vi "pp2_log_state.vi"(8 "Log memo?":bool, 10 "refnum in":refnum<file>, 11 "State In":T1={"Curr  tr"=0, "Curr (ms)"=0, "Cum (ms)"=0, "Run loop diff"=0, "Tone countdown (ms)"=0, "Countdown (ms)"=0, "Curr State"=enum."0 NULL", "Prev State"=enum."1 Habituation", "Null"=FALSE, "Sw"=FALSE, "Tone\nGate"=FALSE, "Stim"=FALSE, "Current DAQ DO Int"=0, "Current Loaded Trial"={"Trial Type Number"=1, "Trial Type"=enum."GO", "Trial Weight"=100, "Shock (mA)"=0.3, "Duration (ms)"=0.25, "Sound Type"=enum."04 FM Sweep", "Stim P1"=4000.0, "Stim P2"=0.0, "Stim P3"=0.0, "Stim P4"=2000.0}, "Next Trial (for display purposes)"={"Trial Type Number"=1, "Trial Type"=enum."GO", "Trial Weight"=100, "Shock (mA)"=0.3, "Duration (ms)"=0.25, "Sound Type"=enum."04 FM Sweep", "Stim P1"=4000.0, "Stim P2"=0.0, "Stim P3"=0.0, "Stim P4"=2000.0}, "Total trials memo"=0, "State start cum memo (ms)"=0, "Last dur jump time memo (ms)"=0, "Last dur shock time memo (ms)"=0, "Tone repeat memo (ms)"=0, "Webcam on"=FALSE, "Webcam recording"=FALSE} {"Current DAQ DO Int" format="%b"; "Next Trial (for display purposes)"."Shock (mA)" min=-1.0 max=5.0; "Next Trial (for display purposes)"."Trial Weight" step=1; "Next Trial (for display purposes)"."Duration (ms)" min=0.0 max=1.0; "Next Trial (for display purposes)"."Trial Type Number" min=1 step=1; "Current Loaded Trial"."Shock (mA)" min=-1.0 max=5.0; "Current Loaded Trial"."Trial Weight" step=1; "Current Loaded Trial"."Duration (ms)" min=0.0 max=1.0; "Current Loaded Trial"."Trial Type Number" min=1 step=1}) -> (2 "refnum out":refnum<file>)   [LabVIEW 2013]
uses:
  pp2_CTL_StateInfo.ctl
  pp2_CTL_State.ctl
  pp2_Trial.ctl
  pp2_CTL_TrialType.ctl
  labolabo2/waveforms/WFTypes.ctl
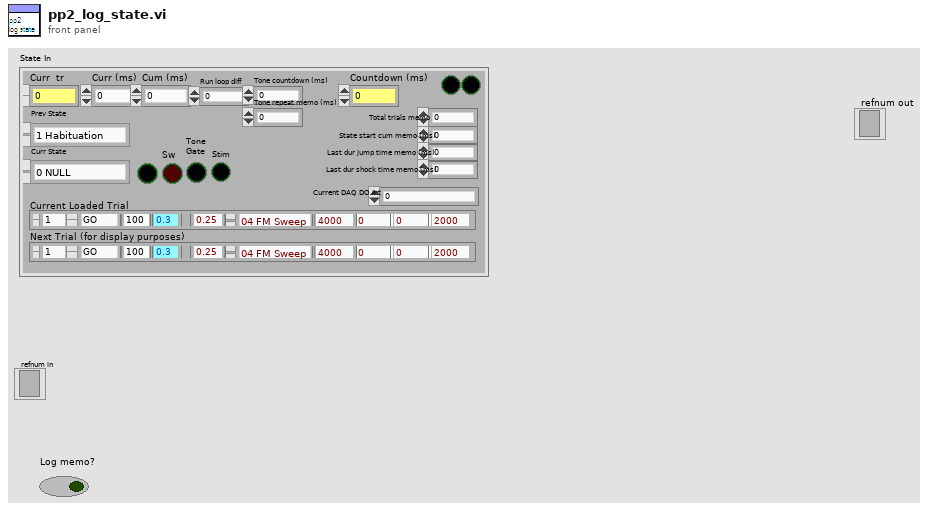
[diagram p1: front panel]
types:
  T1 = typedef "pp2_CTL_StateInfo.ctl" = cluster{"Curr  tr":u16, "Curr (ms)":u32, "Cum (ms)":i64, "Run loop diff":i64, "Tone countdown (ms)":i64, "Countdown (ms)":i64, "Curr State":T2, "Prev State":T2, "Null":bool, "Sw":bool, "Tone\nGate":bool, "Stim":bool, "Current DAQ DO Int":u16, "Current Loaded Trial":T3, "Next Trial (for display purposes)":T3, "Total trials memo":i64, "State start cum memo (ms)":i64, "Last dur jump time memo (ms)":i64, "Last dur shock time memo (ms)":i64, "Tone repeat memo (ms)":i64, "Webcam on":bool, "Webcam recording":bool}
  T2 = typedef "pp2_CTL_State.ctl" = enum8{"0 NULL", "1 Habituation", "2 (Load Trial)", "3 Stay Period", "4 Load Audio/Click Delay", "5 GO Trial", "6 GO Jumped", "7 GO Timeout", "8 NOGO Trial", "9 NOGO Jumped", "10 NOGO Timeout", "11 TEST Trial", "12 TEST Jumped", "13 TEST Timeout", "14 Intertrial Interval", "15 Done"}
  T3 = typedef "pp2_Trial.ctl" = cluster{"Trial Type Number":u8, "Trial Type":T4, "Trial Weight":u32, "Shock (mA)":dbl, "Duration (ms)":dbl, "Sound Type":T5, "Stim P1":dbl, "Stim P2":dbl, "Stim P3":dbl, "Stim P4":dbl}
  T4 = typedef "pp2_CTL_TrialType.ctl" = enum16{"OFF", "GO", "NOGO", "TEST"}
  T5 = typedef "WFTypes.ctl" = enum16{"00 NULL", "01 DC", "02 Noise", "03 Pure Tone", "04 FM Sweep"}
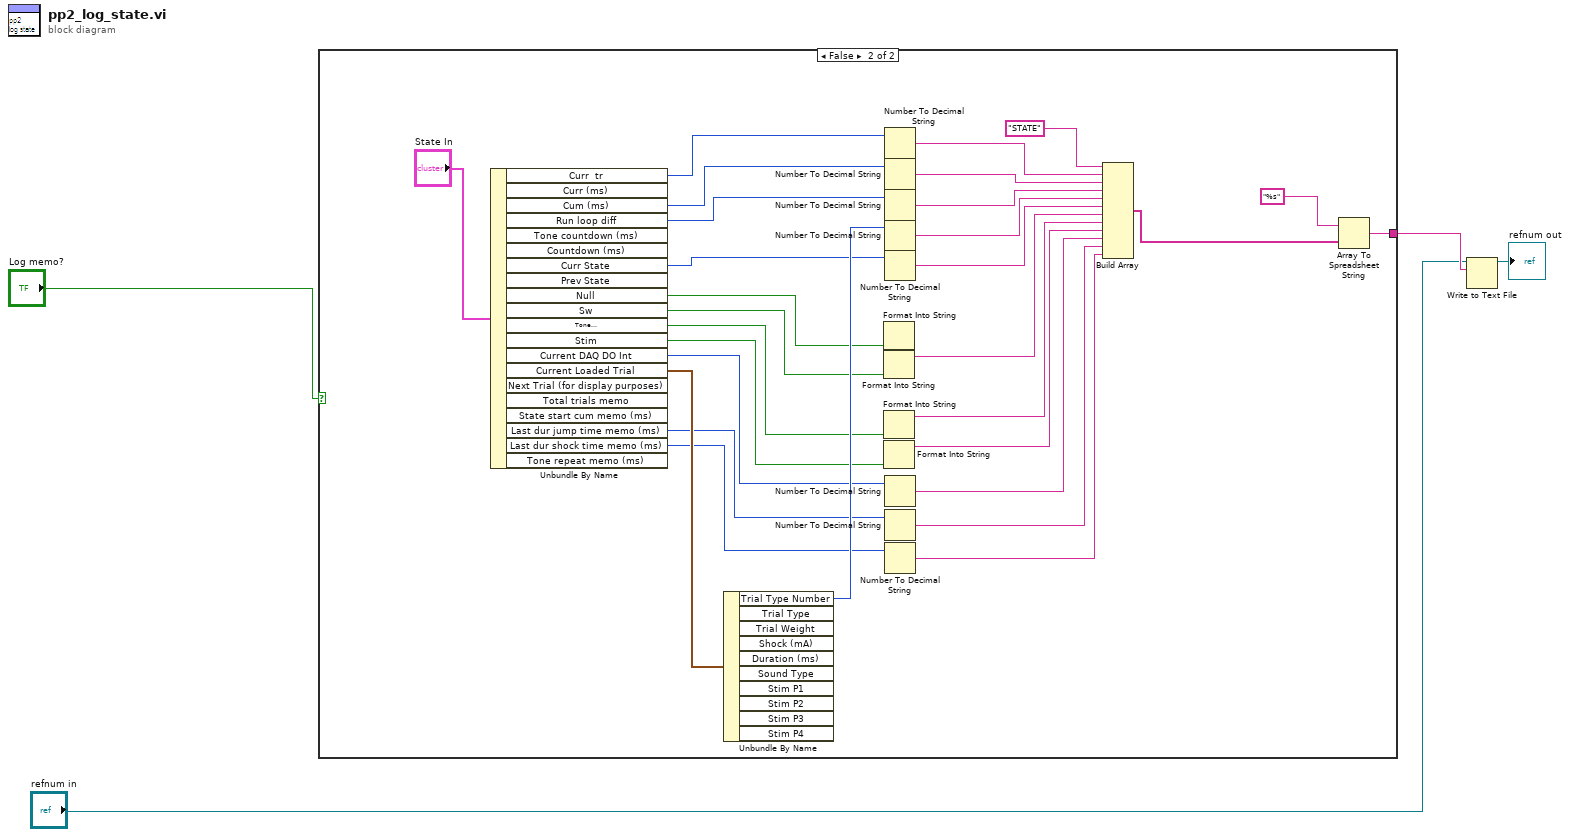
[diagram p0: block diagram]
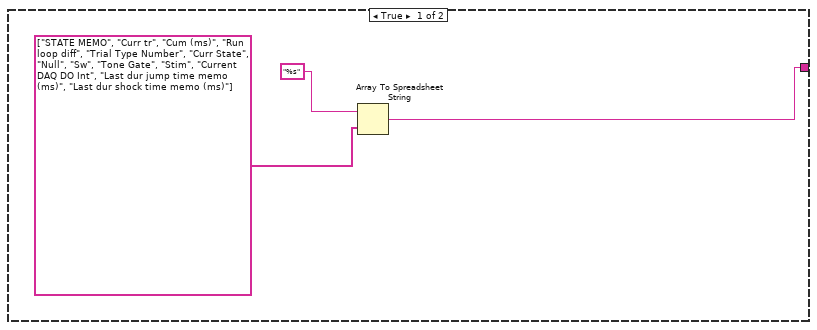
[diagram p2: hidden frame]
diagram:
  n1 = case shown="False" "Log memo?" {
    tunnel: [w5 w29] -> w4
    frame True {
      n2 = Array To Spreadsheet String(array=string[] ["STATE MEMO", "Curr tr", "Cum (ms)", "Run loop diff", "Trial Type Number", "Curr State", "Null", "Sw", "Tone Gate", "Stim", "Current DAQ DO Int", "Last dur jump time memo (ms)", "Last dur shock time memo (ms)"], 3:"%s" ("format string")) -> (spreadsheet string=w5:string)  [unwired: 1 in]
    }
    frame False {
      n3 = Unbundle By Name("State In") -> ("Curr  tr"=w26:u16, "Cum (ms)"=w25:i64, "Run loop diff"=w24:i64, "Curr State"=w21:T2, "Null"=w20:bool, "Sw"=w19:bool, "Tone\nGate"=w18:bool, "Stim"=w17:bool, "Current DAQ DO Int"=w8:u16, "Current Loaded Trial"=w23:T3, "Last dur jump time memo (ms)"=w13:i64, "Last dur shock time memo (ms)"=w12:i64)  [unwired: 8 out]
      n4 = Unbundle By Name(w23) -> ("Trial Type Number"=w22:u8)  [unwired: 9 out]
      n5 = Format Into String(w20) -> ()  [unwired: 3 in, 2 out]
      n6 = Format Into String(w19) -> (resulting string=w16:string)  [unwired: 3 in, 1 out]
      n7 = Format Into String(w18) -> (resulting string=w15:string)  [unwired: 3 in, 1 out]
      n8 = Format Into String(w17) -> (resulting string=w14:string)  [unwired: 3 in, 1 out]
      n9 = Number To Decimal String(number=w26) -> (decimal integer string=w27:string)  [unwired: 1 in]
      n10 = Number To Decimal String(number=w25) -> (decimal integer string=w35:string)  [unwired: 1 in]
      n11 = Number To Decimal String(number=w24) -> (decimal integer string=w34:string)  [unwired: 1 in]
      n12 = Number To Decimal String(number=w22) -> (decimal integer string=w33:string)  [unwired: 1 in]
      n13 = Number To Decimal String(number=w21) -> (decimal integer string=w32:string)  [unwired: 1 in]
      n14 = Number To Decimal String(number=w8) -> (decimal integer string=w9:string)  [unwired: 1 in]
      n15 = Number To Decimal String(number=w13) -> (decimal integer string=w11:string)  [unwired: 1 in]
      n16 = Number To Decimal String(number=w12) -> (decimal integer string=w10:string)  [unwired: 1 in]
      n17 = Build Array("STATE" ("element"), w27, w35, w34, w33, w32, w16, w15, w14, w9, w11, w10) -> (w30:string[])
      n18 = Array To Spreadsheet String(array=w30, 3:"%s" ("format string")) -> (spreadsheet string=w29:string)  [unwired: 1 in]
    }
  }
  n19 = Write to Text File(file (use dialog)="refnum in", text=w4) -> (refnum out=→"refnum out":refnum<file>)  [unwired: 2 in, 2 out]
